vi "Read.vi"(8 "error in":errorcluster, 11 "Megger cluster in":T1={"Read data"={"Firmware version"="", "Model number"="", "Serial number"=0, "Ramp rate"=0.0, "Test Voltage"=0.0, "Test duration"=0.0, "Test stop watch"=0.0, "measured Current (nA)"=0.0, "calculated Resistance"=0.0, "Test Mode"=enum."Insulation resistance (IR)", "Test status"=enum."Waiting to start test"}, "Connected?"=FALSE, "Device status array"=[]}) -> (0 "error out":errorcluster, 3 "Megger cluster out":T1={"Read data"={"Firmware version"="", "Model number"="", "Serial number"=0, "Ramp rate"=0.0, "Test Voltage"=0.0, "Test duration"=0.0, "Test stop watch"=0.0, "measured Current (nA)"=0.0, "calculated Resistance"=0.0, "Test Mode"=enum."Insulation resistance (IR)", "Test status"=enum."Waiting to start test"}, "Connected?"=FALSE, "Device status array"=[]})   [LabVIEW 2014]
doc: "This VI polls the device every half second for data and returns it in a cluster. Run this VI every 10ms, a timer is used internally to control exact timing."
uses:
  Private/Controls/Megger cluster.ctl
  Private/Controls/Global Megger.vi
  Stopwatch/Stop watch/Stop watch.lvlib
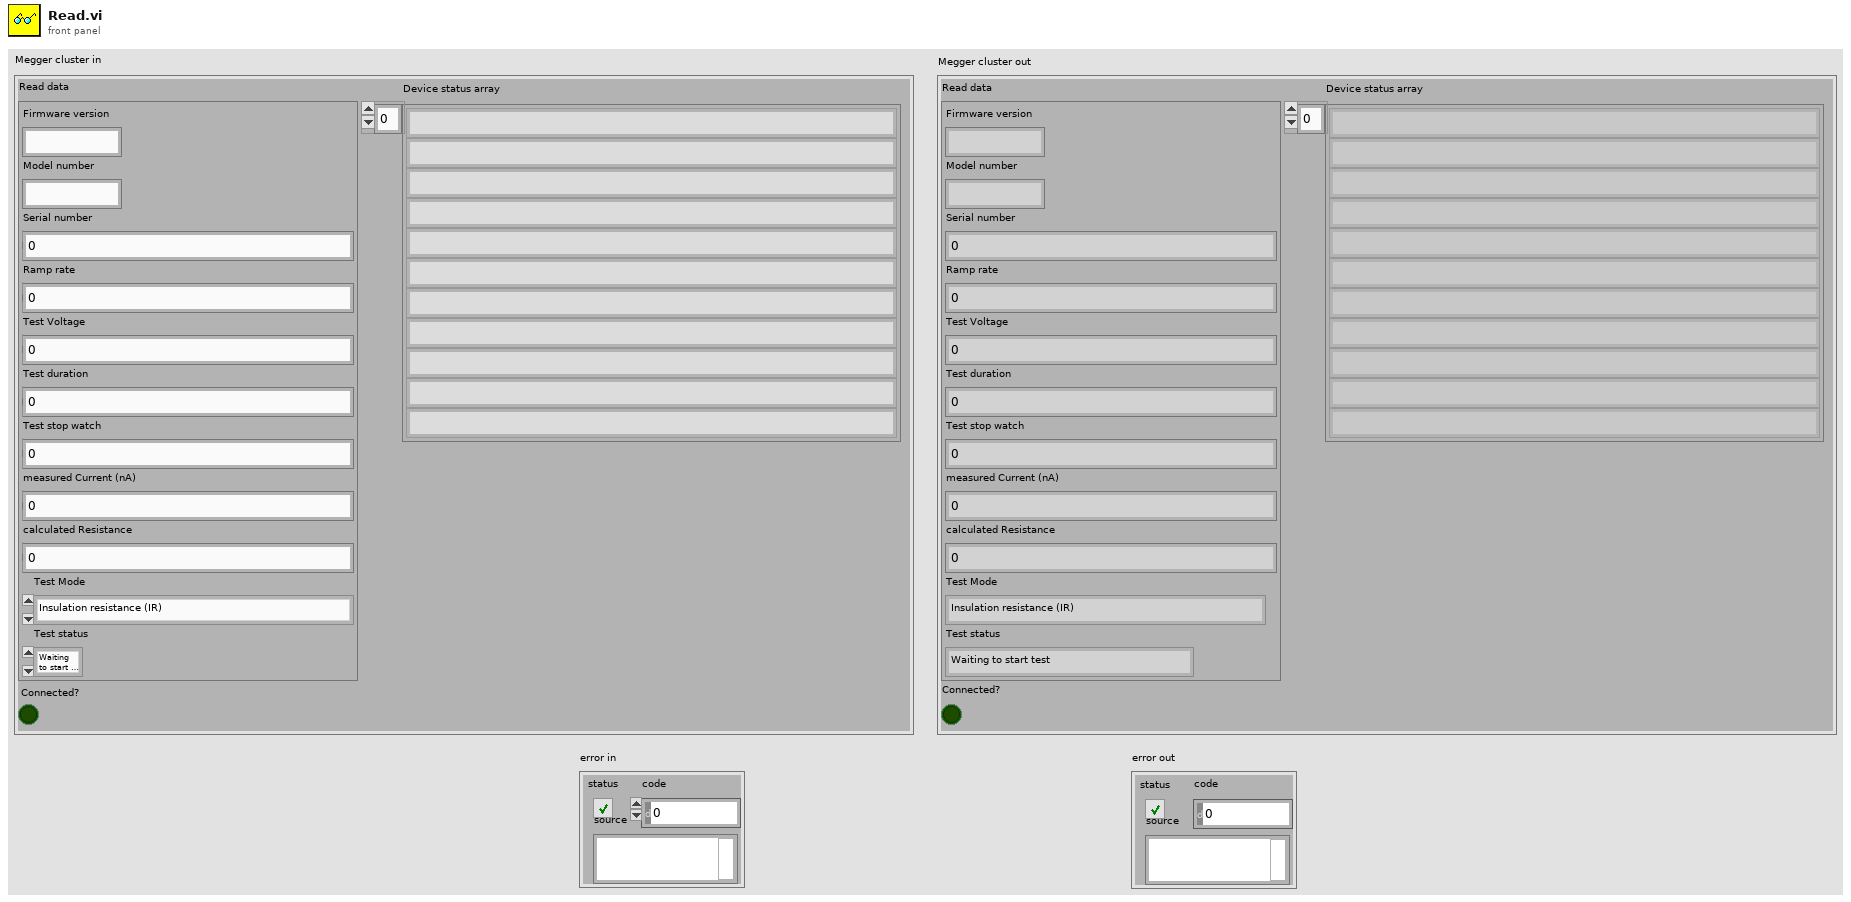
[diagram p1: front panel]
types:
  T1 = typedef "Megger cluster.ctl" = cluster{"Read data":cluster{"Firmware version":string, "Model number":string, "Serial number":i32, "Ramp rate":dbl, "Test Voltage":dbl, "Test duration":sgl, "Test stop watch":sgl, "measured Current (nA)":dbl, "calculated Resistance":dbl, "Test Mode":enum16{"N/A", "Insulation resistance (IR)", "Timed Insulation resistance (IR(t))", "Diaelectric Absorption Ratio (DAR)", "Polarisation Index (PI)", "Diaelectric Dishcharge (DD)", "Step voltage (SV)", "Ramp test (Ramp)"}, "Test status":enum16{"Waiting to start test", "Unable to start test", "Test progressing normally", "Performing post test measurements", "Test has ended normally", "Test has been aborted"}}, "Connected?":bool, "Device status array":string[]}
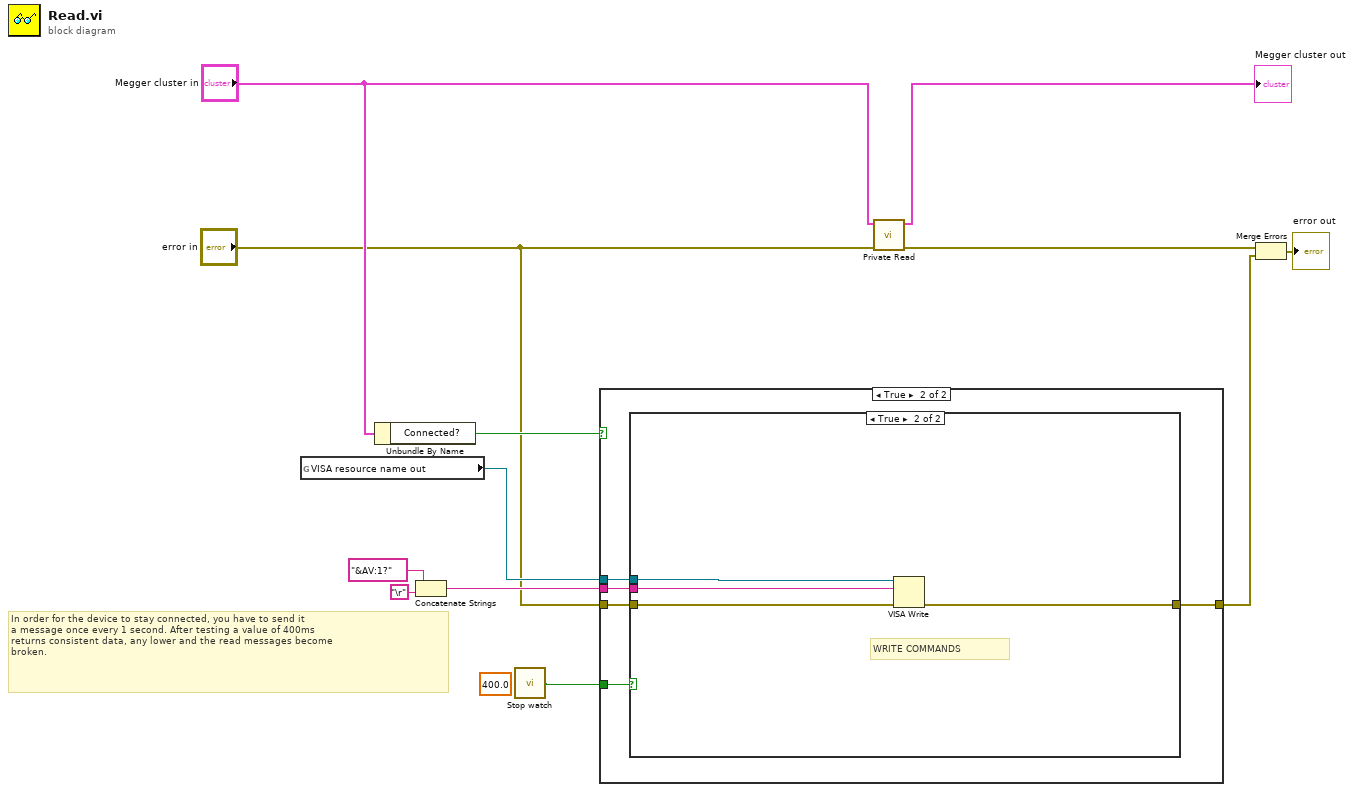
[diagram p0: block diagram]
diagram:
  (unwired) 400.0 ("Time to wait, mS")
  # "In order for the device to stay connected, you have to send it\na message once every 1 second. After testing a value of 400ms\nreturns consistent data, any lower and the read messages become\nbroken."
  n1 = global read "Global Megger.vi" "VISA resource name out"() -> (w10:refnum<visa-resource-name>)
  n2 = Unbundle By Name("Megger cluster in") -> ("Connected?"=w6:bool)
  n3 = Concatenate Strings("&AV:1?" ("write buffer"), "\r") -> (w5:string)
  n4 = call "Stop watch.vi"() -> ("Timer up"=w1:bool)  [unwired: 14 in, 1 out]
  n5 = case shown="True" w6 {
    tunnel: "error in" -> [w13 w18]
    tunnel: w10 -> [_ w17]
    tunnel: [w13 w14] -> w8
    tunnel: w5 -> [_ w16]
    tunnel: w1 -> [_ w15]
    frame False {
    }
    frame True {
      n6 = case shown="True" w15 {
        tunnel: w18 -> [w19 w23]
        tunnel: w17 -> [_ w22]
        tunnel: w16 -> [_ w21]
        tunnel: [w19 w20] -> w14
        frame False {
        }
        frame True {
          # "WRITE COMMANDS"
          n7 = VISA Write(VISA resource name=w22, write buffer=w21, error in (no error)=w23) -> (error out=w20:errorcluster)  [unwired: 2 out]
        }
      }
    }
  }
  n8 = call "Private Read.vi"("error in"="error in", "Megger cluster in"="Megger cluster in") -> ("error out"=w2:errorcluster, "Megger cluster out"=→"Megger cluster out":T1)  [unwired: 7 in, 1 out]
  n9 = Merge Errors(w2, w8) -> (→"error out":errorcluster)
